vi "Constructor.vi"(8 "error in (no error)":errorcluster, 11 "Operation Complete Caller in":refnum<class "Operation Complete Caller.lvclass">) -> (0 "error out":errorcluster, 3 "Operation Complete Caller out":refnum<class "Operation Complete Caller.lvclass">)   [LabVIEW 2022 SP3, in "Operation Complete Caller.lvclass"]
uses:
  Operation Complete Caller.lvclass
  Operation Complete Caller.lvclass/Operation Complete Caller.ctl
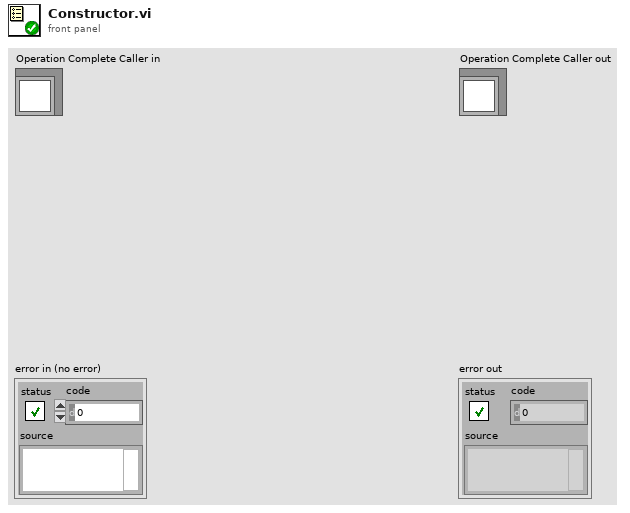
[diagram p1: front panel]
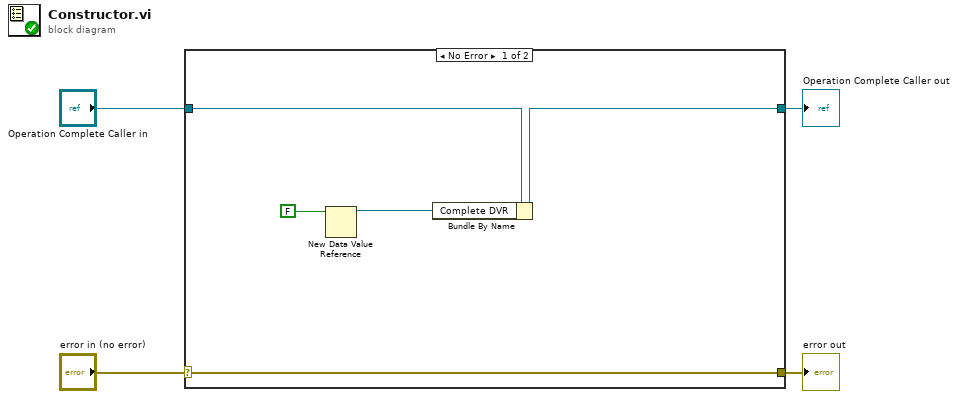
[diagram p0: block diagram]
diagram:
  n1 = case shown="No Error" "error in (no error)" {
    selector: "error in (no error)" -> [w9 w11]
    tunnel: [w9 w11] -> w3
    tunnel: [w5 w10] -> w1
    tunnel: "Operation Complete Caller in" -> [w7 w10]
    frame No Error {
      n2 = New Data Value Reference(data value=FALSE) -> (data value reference=w6:refnum<data-value>)  [unwired: 1 in, 1 out]
      n3 = Bundle By Name(cluster=w7, "Complete DVR"=w6) -> (w5:refnum<class "Operation Complete Caller.lvclass">)
    }
    frame Error {
    }
  }
  "error out" <- w3
  "Operation Complete Caller out" <- w1
